vi "Send Write Actor Filter.vi"(7 "Message Priority (Normal)":T2=enum."Normal", 8 "error in (no error)":errorcluster, 10 "Actor Filter":T1={"PVMonitor"=FALSE, "PVProxy"=FALSE, "GUI"=FALSE, "Other"=TRUE}, 11 "Message Enqueuer":refnum<class "Message Enqueuer.lvclass">) -> (0 "error out":errorcluster, 3 "Message Enqueuer out":refnum<class "Message Enqueuer.lvclass">)   [LabVIEW 2015, in "CS++ObjectManager.lvlib" / "Write Actor Filter Msg.lvclass"]
doc: "Sends the <B>CS++ObjectManager.lvlib:Write Actor Filter Msg.lvclass</B> message.\n\n<B>CS++ObjectManager.lvlib:CS++ObjectManager.lvclass:Write Actor Filter.vi</B> Description:"
uses:
  Write Actor Filter Msg.lvclass
  <vilib>/ActorFramework/Message Enqueuer/Message Enqueuer.lvclass
  <vilib>/ActorFramework/Message Enqueuer/Message Priority.ctl
  Write Actor Filter Msg.lvclass/Write Actor Filter Msg.ctl
  <vilib>/ActorFramework/Message Enqueuer/Message Enqueuer.lvclass/Message Enqueuer.ctl
  <vilib>/ActorFramework/Message Priority Queue/Priority Enqueue.vi
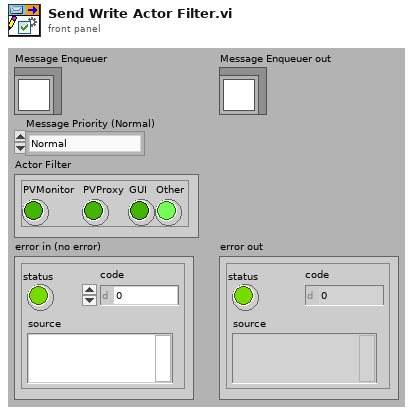
[diagram p1: front panel]
types:
  T1 = cluster{"PVMonitor":bool, "PVProxy":bool, "GUI":bool, "Other":bool}
  T2 = typedef "Actor Framework.lvlib/Message Enqueuer.lvclass/Message Priority.ctl" = enum16{"Low", "Normal", "High"}
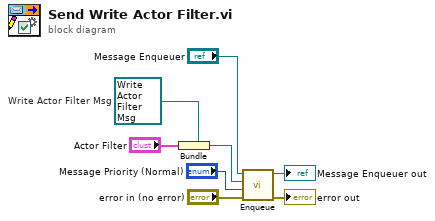
[diagram p0: block diagram]
diagram:
  w2 = refnum<class "Write Actor Filter Msg.lvclass"> refnum  # Write Actor Filter Msg
  n1 = Bundle(cluster=w2, "Actor Filter") -> (w5:refnum<class "Write Actor Filter Msg.lvclass">)
  n2 = call <vilib>:"Enqueue.vi"("error in (no error)"="error in (no error)", "Message Priority (Normal)"="Message Priority (Normal)", "Message"=w5, "Message Enqueuer in"="Message Enqueuer") -> ("error out"=→"error out":errorcluster, "Message Enqueuer out"=→"Message Enqueuer out":refnum<class "Message Enqueuer.lvclass">)  [unwired: 6 in]
